vi "Query Installed modules.vi"(8 "error in":errorcluster, 11 "3300 in":refnum<class "3300.lvclass">) -> (0 "error out":errorcluster, 3 "3300 out":refnum<class "3300.lvclass">)   [LabVIEW 2019, in "3300.lvlib" / "3300.lvclass"]
uses:
  Library/3300.lvclass
  Custom Controls/Modules.ctl
  Library/3300.lvclass/3300.ctl
panel:
  in  "Modules":T1
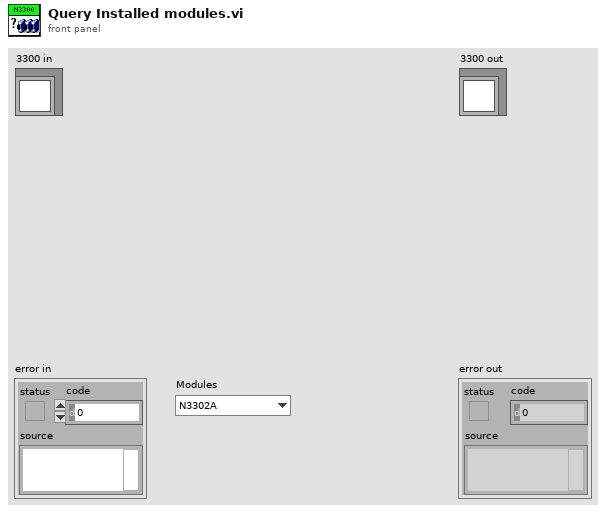
[diagram p1: front panel]
types:
  T1 = typedef "3300.lvlib/3300.lvclass/Modules.ctl" = enum16{"N3302A", "N3303A", "N3304A", "N3305A", "N3306A", "N3307A"}
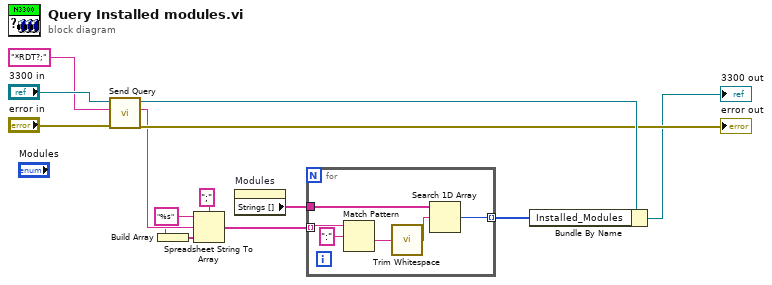
[diagram p0: block diagram]
diagram:
  w3 = "%s" ("format string")
  n1 = call "Send Query.vi"("error in"="error in", "Query"="*RDT?;", "3300 in"="3300 in") -> ("error out"=→"error out":errorcluster, "Read Data"=w5:string, "3300 out"=w10:refnum<class "3300.lvclass">)  [unwired: 6 in]
  n2 = Build Array(w3) -> (w4:string[])
  n3 = Spreadsheet String To Array(delimiter (Tab)=";", format string=w3, spreadsheet string=w5, array type (2D Dbl)=w4) -> (array=w7:string[])
  n4 = property on="Modules" class="Enum (strict)"() -> ("Strings []"=w6:string[])  [unwired: 2 in, 2 out]
  n5 = for {
    tunnel: w7 -> [w19] mode=indexing
    tunnel: w6 -> [w16]
    tunnel: [w14] -> w1 mode=indexing
    n6 = Match Pattern(string=w19, regular expression=":") -> (after substring=w17:string)  [unwired: 1 in, 3 out]
    n7 = call <vilib>:"Trim Whitespace.vi"("string"=w17) -> ("trimmed string"=w15:string)  [unwired: 1 in]
    n8 = Search 1D Array(1D array=w16, element=w15) -> (index of element=w14:i32)  [unwired: 1 in]
  }
  n9 = Bundle By Name(cluster=w10, "Installed_Modules"=w1) -> (→"3300 out":refnum<class "3300.lvclass">)
